vi "BindingQLTY.vi"(4 "错误输入":errorcluster, 6 "总成追溯码":string, 7 "工位追溯码":string) -> (0 "error out":errorcluster)   [LabVIEW 2020]
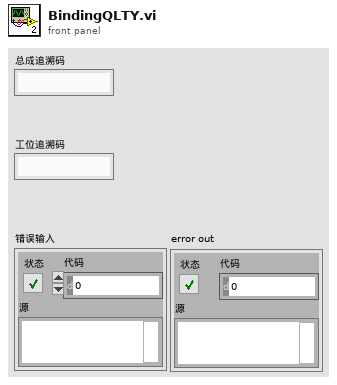
[diagram p1: front panel]
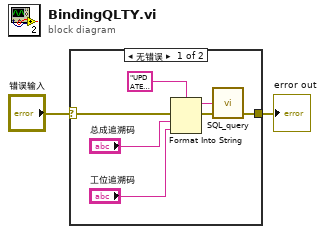
[diagram p0: block diagram]
diagram:
  n1 = case shown="无错误" "错误输入" {
    selector: "错误输入" -> [w6 w10]
    tunnel: [w5 w10] -> w1
    frame No Error {
      n2 = Format Into String(format string="UPDATE [SANLIserver].[dbo].[产品质量2]\nSET [总成追溯码] = N'%s'\nWHERE\n\tdbo.[物料].[工位追溯码] = '%s'", error in=w6, "总成追溯码", "工位追溯码") -> (resulting string=w8:string, error out=w7:errorcluster)  [unwired: 1 in]
      n3 = call "SQL_query.vi"("error in (no error)"=w7, "SQL query"=w8) -> ("error out"=w5:errorcluster)  [unwired: 1 in, 2 out]
    }
    frame Error {
    }
  }
  "error out" <- w1
